vi "GetActivePlayers.vi"(8 "Error In":errorcluster, 11 "XBMC Ref":T1) -> (0 "Error Out":errorcluster, 1 "Response":string, 3 "XBMC Ref":T1)   [LabVIEW 2013, in "LMH-Kodi.lvlib" / "Player.lvlib"]
uses:
  <vilib>/MakerHub/Kodi/Private/Player/Player.lvlib
  Type Defs/XBMC Ref.ctl
  <vilib>/httpClient/ClientHandle.ctl
  Type Defs/ID FGV State.ctl
  Type Defs/Player_GetActivePlayers.ctl
  LMH-Kodi.lvlib
  <vilib>/httpClient/LabVIEWHTTPClient.lvlib
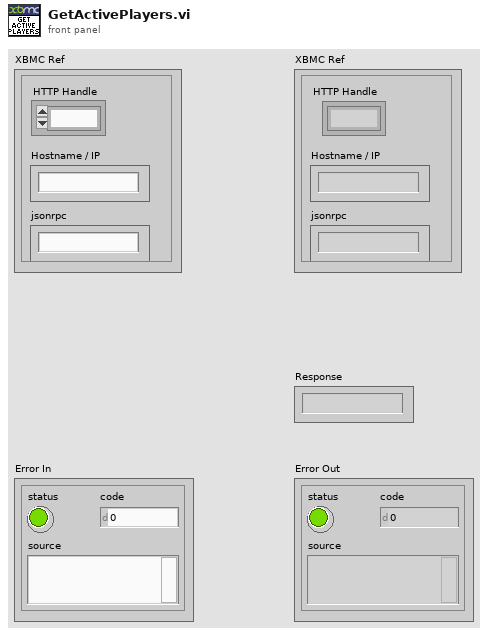
[diagram p1: front panel]
types:
  T1 = typedef "LMH-Kodi.lvlib/XBMC Ref.ctl" = cluster{"HTTP Handle":T2, "Hostname / IP":string, "jsonrpc":string}
  T2 = typedef "LabVIEWHTTPClient.lvlib/ClientHandle.ctl" = refnum<k1>
  T3 = typedef "LMH-Kodi.lvlib/Player.lvlib/Player_GetActivePlayers.ctl" = cluster{"method":string, "jsonrpc":string, "id":i32}
  T4 = enum16{"Player.GetActivePlayers", "Player.GetItem", "Player.GetProperties", "Player.GoTo", "Player.Move", "Player.Open", "Player.PlayPause", "Player.Rotate", "Player.Seek", "Player.SetAudioStream", "Player.SetPartyMode", "Player.SetRepeat", "Player.SetShuffle", "Player.SetSpeed", "Player.SetSubtitle", "Player.Stop", "Player.Zoom"}
  T5 = typedef "LMH-Kodi.lvlib/ID FGV State.ctl" = enum16{"Init", "Peek", "Get++"}
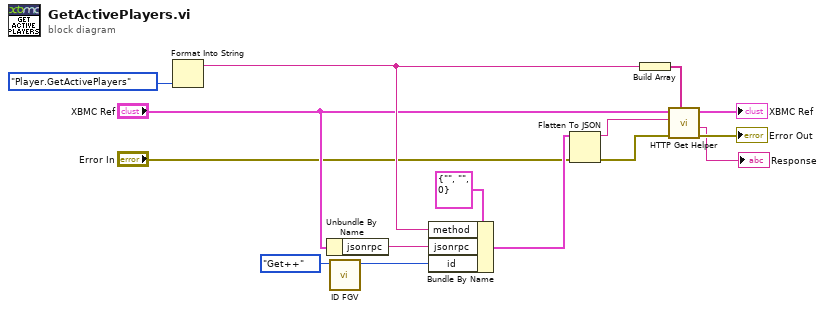
[diagram p0: block diagram]
diagram:
  n1 = Format Into String(T4."Player.GetActivePlayers" ("Method")) -> (resulting string=w11:string)  [unwired: 3 in, 1 out]
  n2 = Unbundle By Name("XBMC Ref") -> ("jsonrpc"=w4:string)
  n3 = call "ID FGV.vi"("FGV State"=ID_FGV_State."Get++") -> ("Value"=w5:i32)  [unwired: 10 in]
  n4 = Bundle By Name(cluster=T3 {"method"="", "jsonrpc"="", "id"=0} ("Player.GetItem"), "method"=w11, "jsonrpc"=w4, "id"=w5) -> (w9:T3)
  n5 = Flatten To JSON(anything=w9, error in (no error)="Error In") -> (JSON string=w8:string, 11:w7:errorcluster)  [unwired: 1 in]
  n6 = Build Array(w11) -> (w12:string[])
  n7 = call "HTTP Get Helper.vi"("Arguments"=w12, "Error In"=w7, "JSON Request"=w8, "XBMC Ref"="XBMC Ref") -> ("Error Out"=→"Error Out":errorcluster, "Response"=→"Response":string, "XBMC Ref"=→"XBMC Ref":T1)  [unwired: 5 in]
